vi "Read FPGA FIFO.vi"(6 "Error In":errorcluster, 9 "Vessel.lvclass":refnum<class "Vessel.lvclass">) -> (0 "Error Out":errorcluster, 3 "Vessel.lvclass 2":refnum<class "Vessel.lvclass">)   [LabVIEW 2014, in "Vessel.lvclass"]
uses:
  Vessel.lvclass
  Vessel.lvclass/Vessel.ctl
  <vilib>/Utility/error.llb/Error Cluster From Error Code.vi
  <vilib>/rvi/errors/niLvFpgaAdjustHostInterfaceError.vi
  <vilib>/rvi/interface/nirviMethod/nirviMethod.xnode
  FPGA Bitfiles/MinervaControlSy_FPGATarget_9870InterfaceDMA_4D1233B8.lvbitx
  cRIO/FPGA/9870 Interface DMA (FPGA).vi
  Supervisor/Supervisor.lvclass
  <vilib>/rvi/errors/niLvFpgaMergeErrorWithErrorCode.vi
  <vilib>/FPGAPlugInAG/cRIO-9074/niLvFpga_ReadFifo_cRIO-9074.vi
panel:
  in  "use chair":bool
  out "UDP error out":errorcluster
  out "APOS NED":dbl[](array[numeric]) format="%#.3f"
  out "kPa":dbl=100000.0 format="%#.1f"
  in  "depth ring":u16(ring)=2 items=["Saiv", "DVL", "Digiquartz"]
  out "DVL":string
  out "MT_BITS":u8[](array[numeric])
  out "Pos_s":dbl[](array[numeric])
  out "Altitudes":dbl[](array[numeric])
  out "Telebuf":u8[](array[numeric])
  out "NAVI OK":string
  out "MT_DATA":sgl[](array[numeric])
  in  "alt off [m]":dbl=0.2
  out "dvl_m":dbl[](array[numeric])
  out "MRU out":dbl[](array[numeric])
  out "Signals out":dbl[](array[numeric]) format="%#.2f"
  out "Elements Remaining\n after read":u32
  # "10."
  # "20."
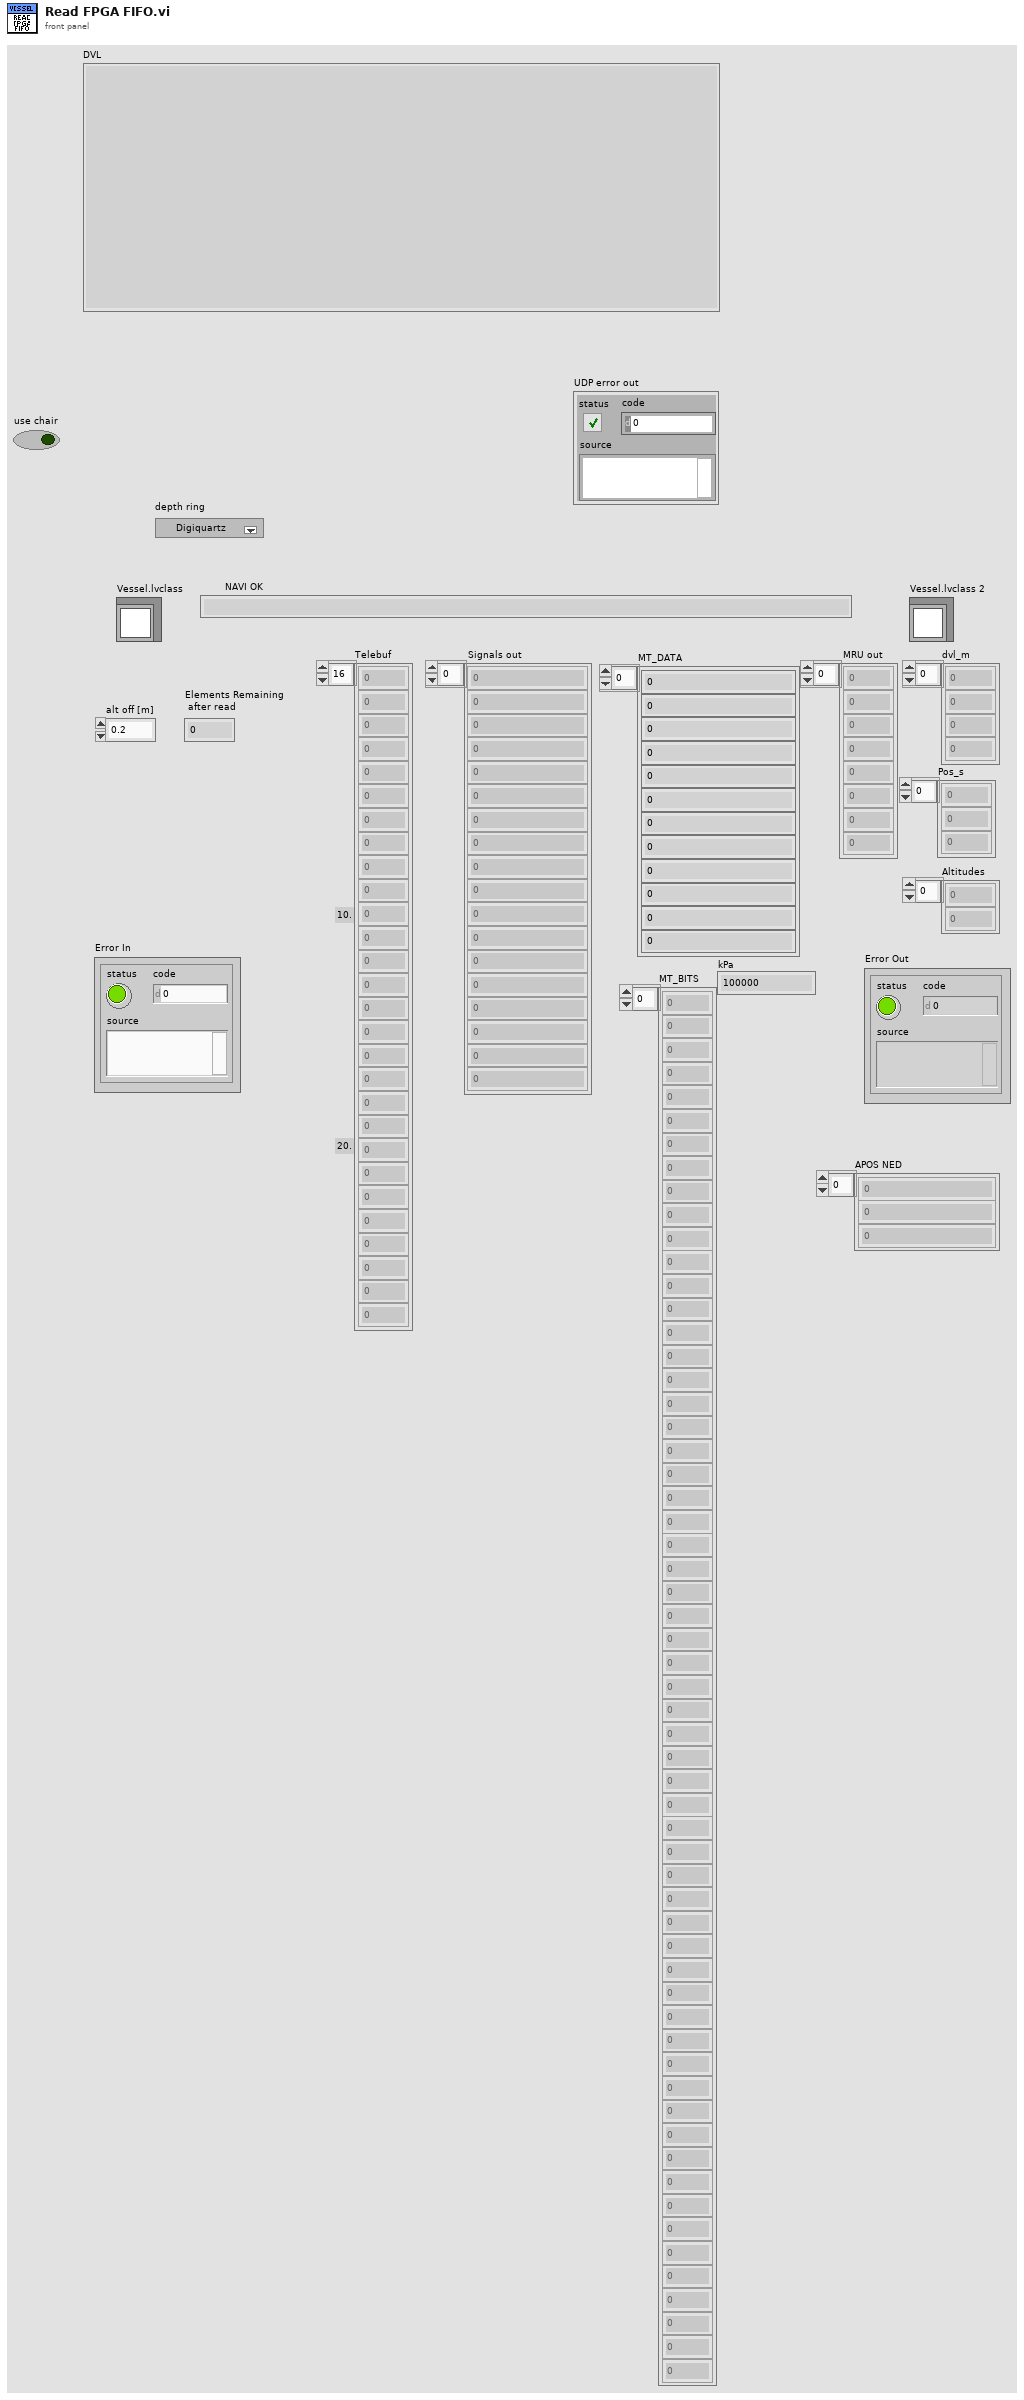
[diagram p1: front panel]
types:
  T1 = typedef "nicrio_cRIO-9871_BaudRateEnum.ctl" = enum16{"75 bps", "110 bps", "134 bps", "150 bps", "300 bps", "600 bps", "1200 bps", "1800 bps", "2400 bps", "4800 bps", "7200 bps", "9600 bps", "14.4 kbps", "19.2 kbps", "28.8 kbps", "38.4 kbps", "57.6 kbps", "115.2 kbps", "230.4 kbps", "460.8 kbps", "921.6 kbps"}
  T2 = typedef "nicrio_cRIO-9871_DataBitsEnum.ctl" = enum8{"5", "6", "7", "8"}
  T3 = typedef "nicrio_cRIO-9871_ParityEnum.ctl" = enum8{"None", "Odd", "Even", "Mark", "Space"}
  T4 = typedef "nicrio_cRIO-9871_StopBitsEnum.ctl" = enum8{"1", "1.5", "2"}
  T5 = typedef "nicrio_cRIO-9871_FlowControlEnum.ctl" = enum8{"None", "Software (XON / XOFF)", "Hardware (RTS / CTS)"}
  T6 = cluster{"Baud Rate":T1, "Data Bits":T2, "Parity":T3, "Stop Bits":T4, "Flow Control":T5}[]
  T7 = cluster{"Axis Translation":cluster{"X-Axis":dbl, "Y-Axis":dbl, "Z-Axis":dbl}, "Axis Rotation":cluster{"X-Axis":dbl, "Y-Axis":dbl, "Z-Axis":dbl}}
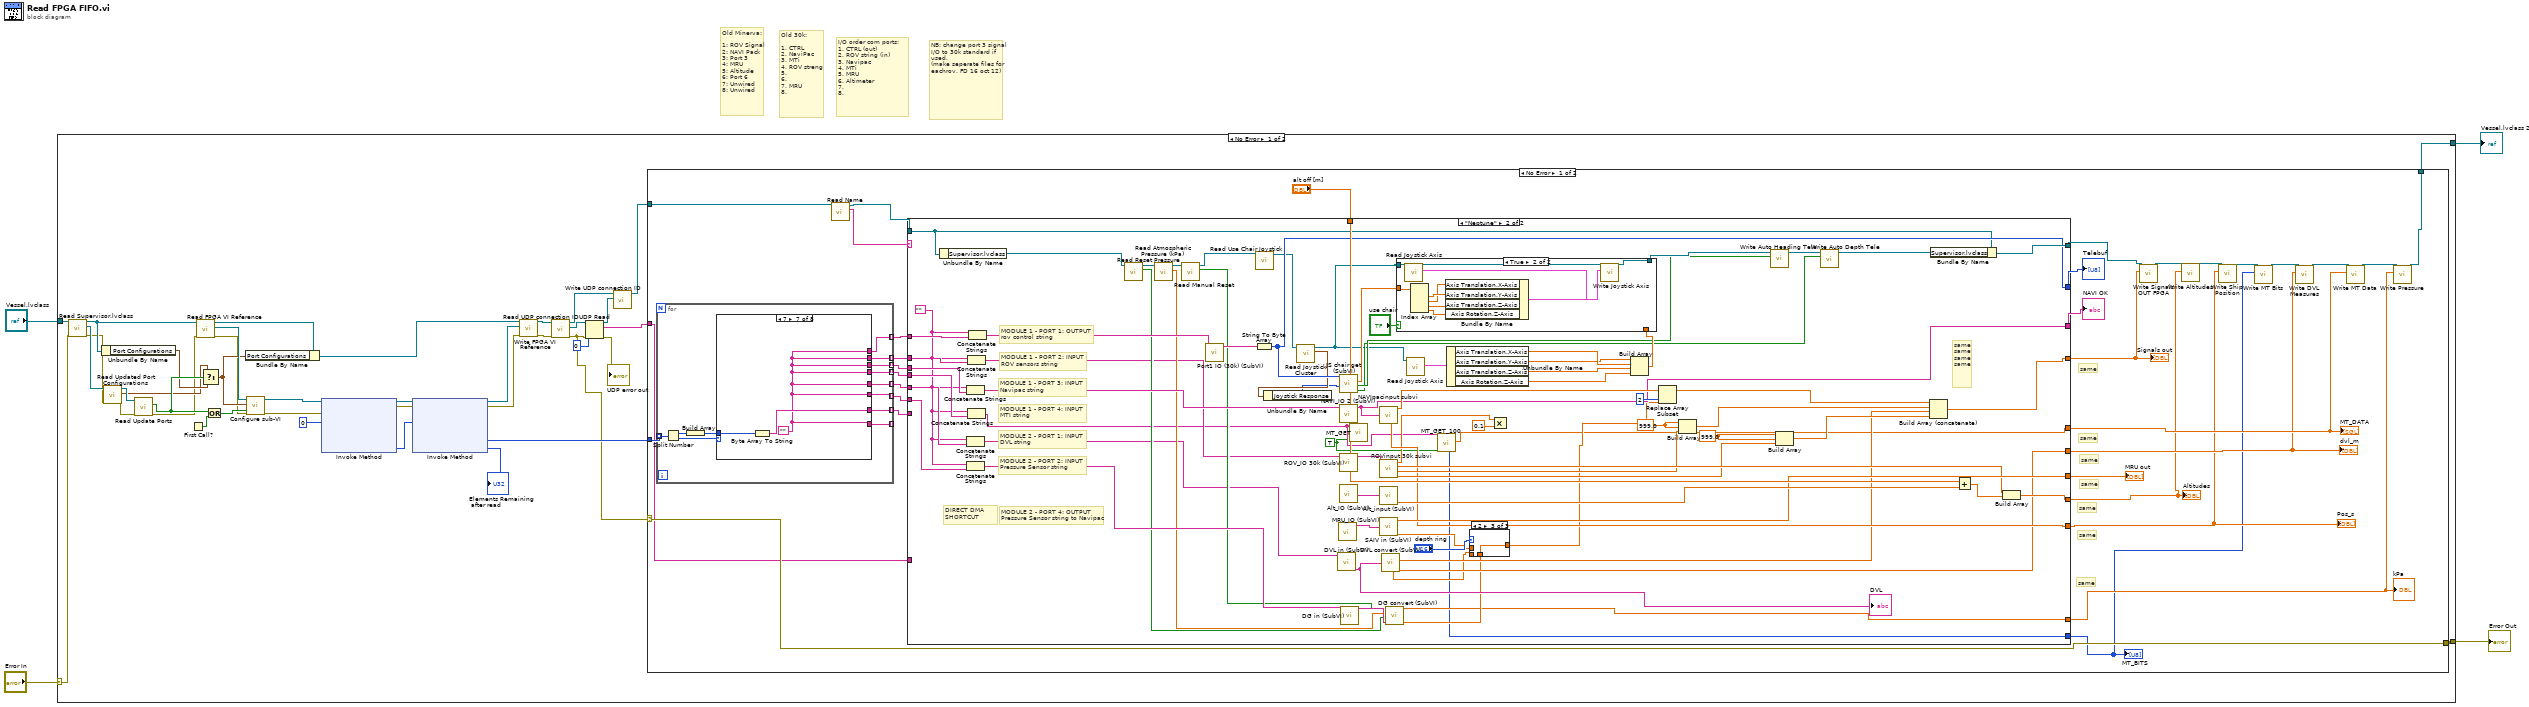
[diagram p0: block diagram]
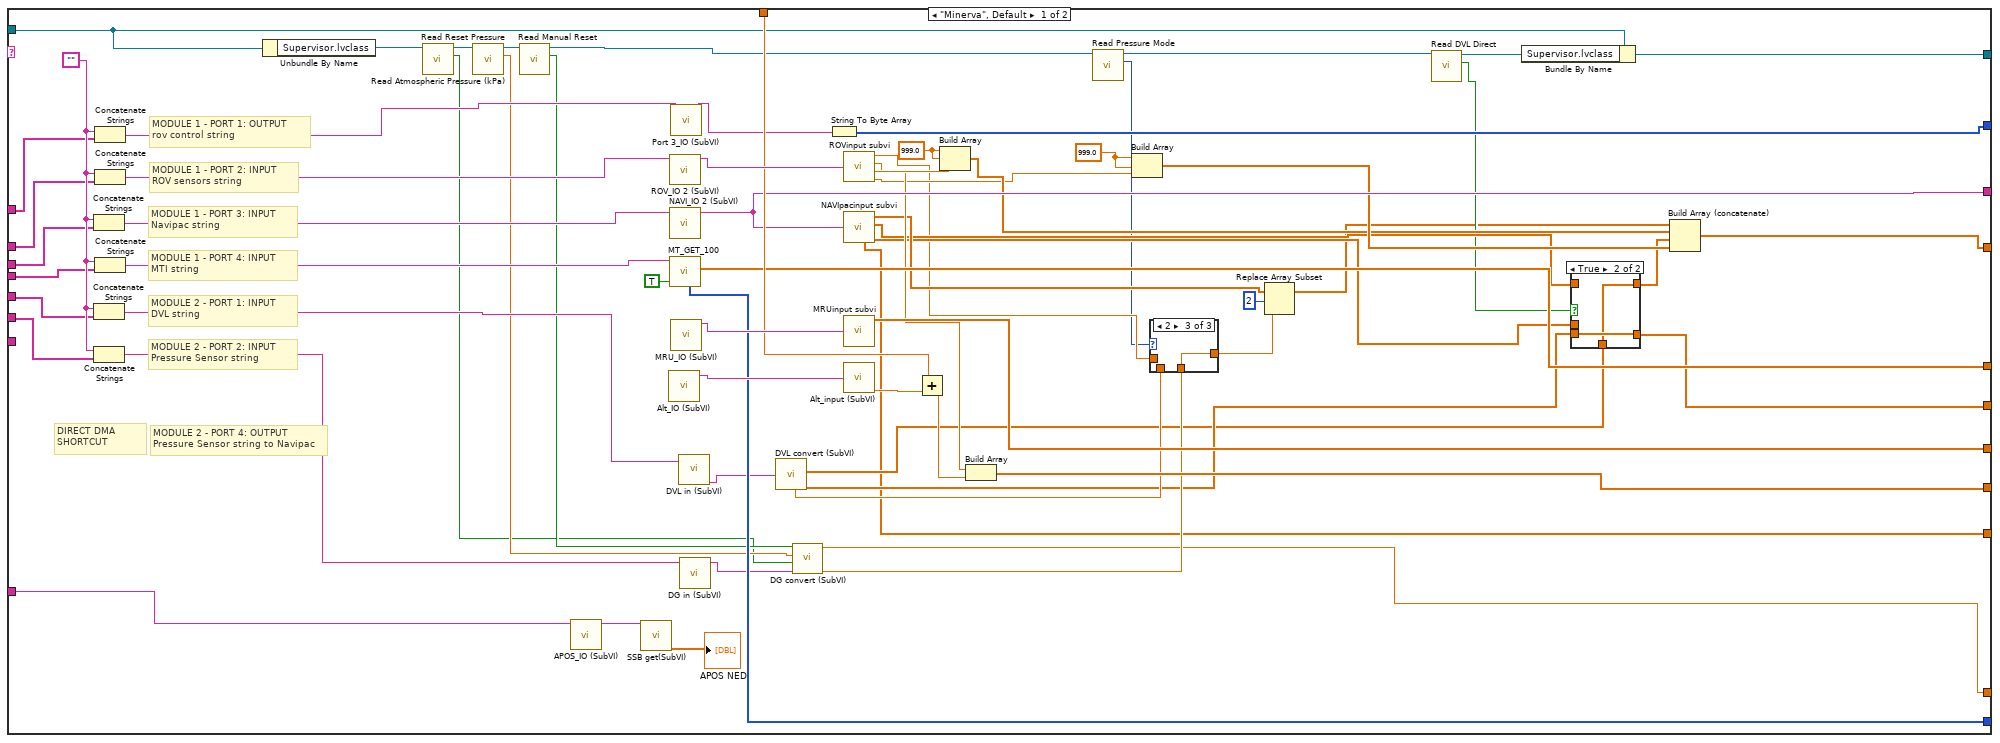
[diagram p2: hidden frame]
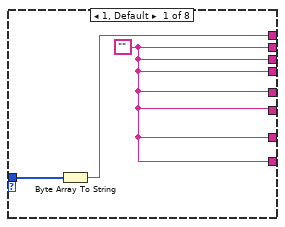
[diagram p9: hidden frame]
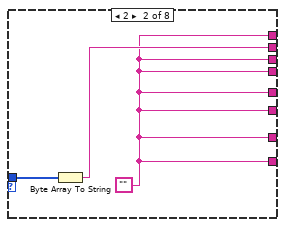
[diagram p10: hidden frame]
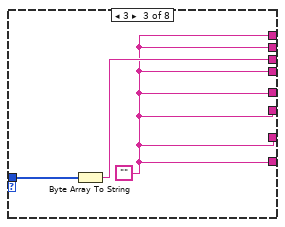
[diagram p11: hidden frame]
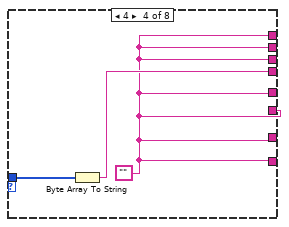
[diagram p12: hidden frame]
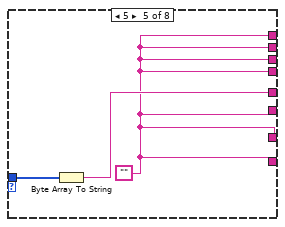
[diagram p13: hidden frame]
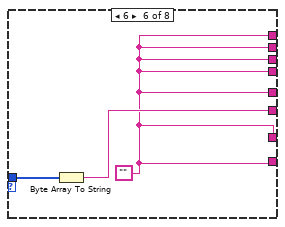
[diagram p14: hidden frame]
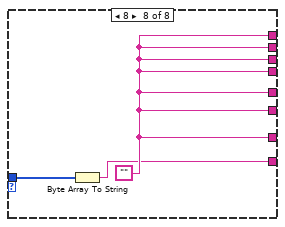
[diagram p15: hidden frame]
diagram:
  # "NB: change port 3 signal I/O to 30k standard if used. \n(make seperate files for eachrov, FD 16 oct 12)"
  # "I/O order com ports:\n1. CTRL (out)\n2. ROV string (in)\n3. Navipac\n4. MTi\n5. MRU\n6. Altimeter\n7. \n8."
  # "Old 30k:\n\n1. CTRL\n2. NaviPac\n3. MTi\n4. ROV streng\n5.\n6.\n7. MRU\n8."
  # "Old Minerva:\n\n1: ROV Signal\n2: NAVI Pack\n3: Port 3\n4: MRU\n5: Altitude \n6: Port 6\n7: Unwired\n8: Unwired"
  n1 = case shown="No Error" "Error In" {
    selector: "Error In" -> [w10 w281]
    tunnel: "Vessel.lvclass" -> [w33 w282]
    tunnel: [w36 w281] -> w2
    tunnel: [w22 w282] -> w1
    frame No Error {
      n2 = call "Read Supervisor.lvclass.vi"("error in (no error)"=w10, "Vessel in"=w33) -> ("error out"=w9:errorcluster, "Supervisor.lvclass"=w32:refnum<class "Supervisor.lvclass">, "Vessel out"=w28:refnum<class "Vessel.lvclass">)  [unwired: 7 in]
      n3 = Unbundle By Name(w28) -> ("Port Configurations"=w26:T6)
      n4 = call-dynamic "Read Updated Port Configurations.vi"("error in (no error)"=w9, "Supervisor in"=w32) -> ("error out"=w8:errorcluster, "Updated Port Configurations"=w25:T6, "Supervisor out"=w31:refnum<class "Supervisor.lvclass">)  [unwired: 7 in]
      n5 = call-dynamic "Read Update Ports.vi"("error in (no error)"=w8, "Supervisor in"=w31) -> ("error out"=w7:errorcluster, "Update Ports"=w27:bool)  [unwired: 7 in, 1 out]
      n6 = First Call?() -> (First Call?: T/F=w30:bool)
      n7 = call-dynamic "Read FPGA VI Reference.vi"("error in (no error)"=w7, "Vessel in"=w28) -> ("error out"=w6:errorcluster, "FPGA VI Reference Out"=w35:refnum<k20>, "Vessel out"=w24:refnum<class "Vessel.lvclass">)  [unwired: 7 in]
      n8 = Select(t=w25, s=w27, f=w26) -> (s? t:f=w23:T6)
      n9 = Or(x=w27, y=w30) -> (x .or. y?=w29:bool)
      n10 = Bundle By Name(cluster=w24, "Port Configurations"=w23) -> (w21:refnum<class "Vessel.lvclass">)
      n11 = call "Configure sub-VI.vi"("error in"=w6, "Update Config"=w29, "Port Configurations"=w23, "FPGA VI Reference In"=w35) -> ("error out"=w5:errorcluster, "FPGA VI Reference Out"=w34:refnum<k20>)  [unwired: 6 in]
      n12 = xnode "Invoke Method"("FPGA VI Reference In"=w34, "error in"=w5, "Number of Elements"=u32 0) -> ("FPGA VI Reference Out"=w41:refnum<k20>, "error out"=w42:errorcluster, "Elements Remaining"=w44:u32)  [unwired: 1 in, 1 out]
      n13 = xnode "Invoke Method"("FPGA VI Reference In"=w41, "error in"=w42, "Number of Elements"=w44) -> ("FPGA VI Reference Out"=w38:refnum<k20>, "error out"=w37:errorcluster, "Data"=w40:u16[], "Elements Remaining"=→"Elements Remaining\n after read":u32)  [unwired: 1 in]
      n14 = call-dynamic "Write FPGA VI Reference.vi"("error in (no error)"=w37, "FPGA VI Reference Out 2"=w38, "Vessel in"=w21) -> ("error out"=w18:errorcluster, "Vessel out"=w19:refnum<class "Vessel.lvclass">)  [unwired: 7 in]
      n15 = call-dynamic "Read UDP connection ID.vi"("error in (no error)"=w18, "Vessel in"=w19) -> ("error out"=w13:errorcluster, "UDP connection ID"=w20:refnum<k16>, "Vessel out"=w16:refnum<class "Vessel.lvclass">)  [unwired: 7 in]
      n16 = UDP Read(connection ID=w20, timeout ms (25000)=0, 8:w13) -> (data out=w17:string, error out=→"UDP error out":errorcluster, 3:w14:refnum<k16>)  [unwired: 1 in, 2 out]
      n17 = call-dynamic "Write UDP connection ID.vi"("UDP connection ID"=w14, "Vessel in"=w16) -> ("Vessel out"=w15:refnum<class "Vessel.lvclass">)  [unwired: 8 in, 1 out]
      n18 = case shown="No Error" w13 {
        selector: w13 -> [w71 w280]
        tunnel: w40 -> [w73 _]
        tunnel: [w71 w280] -> w36
        tunnel: w15 -> [w61 w279]
        tunnel: [w59 w279] -> w22
        tunnel: w17 -> [w60 _]
        frame No Error {
          # "same"
          # "same"
          # "same"
          # "same"
          # "same"
          # "same"
          # "same"
          n19 = for {
            tunnel: w73 -> [w248] mode=indexing
            tunnel: [w252] -> w74 mode=indexing
            tunnel: [w251] -> w75 mode=indexing
            tunnel: [w250] -> w69 mode=indexing
            tunnel: [w249] -> w76 mode=indexing
            tunnel: [w246] -> w72 mode=indexing
            tunnel: [w245] -> w68 mode=indexing
            tunnel: [w244] -> w67 mode=indexing
            tunnel: [w243] -> _ mode=indexing
            n20 = Split Number(x=w248) -> (hi(x)=w254:u8, lo(x)=w253:u8)
            n21 = Build Array(w254) -> (w247:u8[])
            n22 = case shown="7" w253 {
              tunnel: [w256 w258 w261 w264 w267 w270 w273 w277] -> w252
              tunnel: [w255 w259 w261 w264 w267 w270 w273 w277] -> w251
              tunnel: [w255 w258 w262 w264 w267 w270 w273 w277] -> w250
              tunnel: [w255 w258 w261 w265 w267 w270 w273 w277] -> w249
              tunnel: w247 -> [w257 w260 w263 w266 w269 w272 w275 w278]
              tunnel: [w255 w258 w261 w264 w268 w270 w273 w277] -> w246
              tunnel: [w255 w258 w261 w264 w267 w271 w273 w277] -> w245
              tunnel: [w255 w258 w261 w264 w267 w270 w274 w277] -> w244
              tunnel: [w255 w258 w261 w264 w267 w270 w273 w276] -> w243
              frame 1, Default {
                w255 = ""
                n23 = Byte Array To String(unsigned byte array=w257) -> (string=w256:string)
              }
              frame 2 {
                w258 = ""
                n24 = Byte Array To String(unsigned byte array=w260) -> (string=w259:string)
              }
              frame 3 {
                w261 = ""
                n25 = Byte Array To String(unsigned byte array=w263) -> (string=w262:string)
              }
              frame 4 {
                w264 = ""
                n26 = Byte Array To String(unsigned byte array=w266) -> (string=w265:string)
              }
              frame 5 {
                w267 = ""
                n27 = Byte Array To String(unsigned byte array=w269) -> (string=w268:string)
              }
              frame 6 {
                w270 = ""
                n28 = Byte Array To String(unsigned byte array=w272) -> (string=w271:string)
              }
              frame 7 {
                w273 = ""
                n29 = Byte Array To String(unsigned byte array=w275) -> (string=w274:string)
              }
              frame 8 {
                w277 = ""
                n30 = Byte Array To String(unsigned byte array=w278) -> (string=w276:string)
              }
            }
          }
          n31 = call-dynamic "Read Name.vi"("Vessel in"=w61) -> ("Name"=w65:string, "Vessel out"=w66:refnum<class "Vessel.lvclass">)  [unwired: 8 in, 1 out]
          n32 = case shown="\"Neptune\"" w65 {
            tunnel: w76 -> [w140 w228]
            tunnel: w75 -> [w142 w227]
            tunnel: w74 -> [w143 w226]
            tunnel: [w120 w186] -> w51
            tunnel: w72 -> [w139 w158]
            tunnel: [w131 w185] -> w70
            tunnel: [w101 w180] -> w54
            tunnel: w69 -> [w141 w222]
            tunnel: w68 -> [w138 w159]
            tunnel: w66 -> [w116 w195]
            tunnel: [w115 w219] -> w52
            tunnel: w67 -> [_ _]
            tunnel: "alt off [m]" -> [w132 w206]
            tunnel: [w130 w205] -> w63
            tunnel: [w127 w155] -> w56
            tunnel: [w128 w204] -> w62
            tunnel: [w117 w196] -> w45
            tunnel: [w79 w184] -> w53
            tunnel: [w113 w154] -> w48
            tunnel: [w95 w171] -> w58
            tunnel: w60 -> [w92 _]
            frame "Minerva", Default {
              w122 = 999.0 ("element")
              w124 = 999.0 ("element")
              w144 = ""
              # "DIRECT DMA SHORTCUT"
              # "MODULE 2 - PORT 4: OUTPUT\nPressure Sensor string to Navipac"
              # "MODULE 2 - PORT 2: INPUT\nPressure Sensor string"
              # "MODULE 2 - PORT 1: INPUT\nDVL string"
              # "MODULE 1 - PORT 4: INPUT\nMTI string"
              # "MODULE 1 - PORT 3: INPUT\nNavipac string"
              # "MODULE 1 - PORT 2: INPUT\nROV sensors string"
              # "MODULE 1 - PORT 1: OUTPUT\nrov control string"
              n33 = Concatenate Strings(w144, w141) -> (w126:string)
              n34 = Concatenate Strings(w144, w139) -> (w93:string)
              n35 = Concatenate Strings(w144, w138) -> (w107:string)
              n36 = Concatenate Strings(w144, w143) -> (w114:string)
              n37 = Concatenate Strings(w144, w142) -> (w94:string)
              n38 = Concatenate Strings(w144, w140) -> (w125:string)
              n39 = Unbundle By Name(w116) -> ("Supervisor.lvclass"=w84:refnum<class "Supervisor.lvclass">)
              n40 = call-dynamic "Read Reset Pressure.vi"("Supervisor in"=w84) -> ("Reset Pressure"=w81:bool, "Supervisor out"=w86:refnum<class "Supervisor.lvclass">)  [unwired: 8 in, 1 out]
              n41 = call-dynamic "Read Atmospheric Pressure (kPa).vi"("Supervisor in"=w86) -> ("Atmospheric Pressure (deciBar)"=w82:dbl, "Supervisor out"=w85:refnum<class "Supervisor.lvclass">)  [unwired: 8 in, 1 out]
              n42 = call-dynamic "Read Manual Reset.vi"("Supervisor in"=w85) -> ("Manual Reset"=w83:bool, "Supervisor out"=w77:refnum<class "Supervisor.lvclass">)  [unwired: 8 in, 1 out]
              n43 = call "APOS_IO (SubVI).vi"("GPS in"=w92) -> ("GPS OK"=w91:string)  [unwired: 9 in, 1 out]
              n44 = call "SSB get(SubVI).vi"("String"=w91) -> ("APOS NED"=→"APOS NED":dbl[])  [unwired: 4 in, 1 out]
              n45 = call "Alt_IO (SubVI).vi"() -> ("Altimeter OK"=w135:string)  [unwired: 11 in]
              n46 = call "ROV_IO 2 (SubVI).vi"("ROV string"=w94) -> ("ROV OK"=w137:string)  [unwired: 10 in]
              n47 = call "NAVI_IO 2 (SubVI).vi"("NAVI string"=w126) -> ("NAVI OK"=w131:string)  [unwired: 10 in]
              n48 = call "MT_GET_100.vi"("Use checksum"=TRUE, "read buffer"=w125) -> ("MT_DATA"=w127:sgl[], "MT_BITS"=w113:u8[])  [unwired: 6 in, 2 out]
              n49 = call "Port 3_IO (SubVI).vi"("port 3 hex  string"=w114) -> ("port 3 OK"=w129:string)  [unwired: 10 in]
              n50 = call "MRU_IO (SubVI).vi"() -> ("MRU OK"=w134:string)  [unwired: 11 in]
              n51 = call "DVL in (SubVI).vi"("DVL string"=w93) -> ("DVL OK"=w111:string)  [unwired: 10 in]
              n52 = call "DG in (SubVI).vi"("DG string"=w107) -> ("DG OK"=w112:string)  [unwired: 10 in]
              n53 = call "DVL convert (SubVI).vi"("String"=w111) -> ("depth"=w105:dbl, "dvl alts"=w102:dbl[], "u_bt_dvl"=w97:dbl[])  [unwired: 1 in, 2 out]
              n54 = call "DG convert (SubVI).vi"("String"=w112, "Reset pressure"=w81, "atm kPa"=w82, "manual reset"=w83) -> ("depth"=w104:dbl, "Pressure (deciBAR = 10*kPASCAL)"=w95:dbl)  [unwired: 1 in, 1 out]
              n55 = String To Byte Array(string=w129) -> (unsigned byte array=w128:u8[])
              n56 = call "ROVinput subvi.vi"("String"=w137) -> ("depth"=w96:dbl, "altitude"=w119:dbl, "heading"=w123:dbl, "yaw rate"=w106:dbl)
              n57 = call "NAVIpacinput subvi.vi"("String"=w131) -> ("Pos_s"=w79:dbl[], "a_dvl"=w100:dbl[], "vb_dvl"=w99:dbl[], "NED_tp"=w110:dbl[])  [unwired: 2 out]
              n58 = call "MRUinput subvi.vi"("String"=w134) -> ("MRU out"=w130:dbl[])  [unwired: 3 in]
              n59 = call "Alt_input (SubVI).vi"("String"=w135) -> ("altitude"=w133:dbl)  [unwired: 3 in]
              n60 = Add(x=w132, y=w133) -> (x+y=w118:dbl)
              n61 = Build Array(w124, w124, w123) -> (w108:dbl[])
              n62 = Build Array(w119, w118) -> (w117:dbl[])
              n63 = call-dynamic "Read Pressure Mode.vi"("Supervisor in"=w77) -> ("Pressure Mode"=w87:i16, "Supervisor out"=w80:refnum<class "Supervisor.lvclass">)  [unwired: 8 in, 1 out]
              n64 = Build Array(w122, w122, w106) -> (w121:dbl[])
              n65 = case shown="2" w87 {
                tunnel: w105 -> [_ w150 _]
                tunnel: [w149 w150 w151] -> w103
                tunnel: w96 -> [w149 _ _]
                tunnel: w104 -> [_ _ w151]
                frame 0, Default {
                }
                frame 1 {
                }
                frame 2 {
                }
              }
              n66 = Replace Array Subset(array=w110, new element=w103, index=2) -> (w78:dbl[])
              n67 = call-dynamic "Read DVL Direct.vi"("Supervisor in"=w80) -> ("DVL Direct"=w88:bool, "Supervisor out"=w89:refnum<class "Supervisor.lvclass">)  [unwired: 8 in, 1 out]
              n68 = Bundle By Name(cluster=w116, "Supervisor.lvclass"=w89) -> (w115:refnum<class "Vessel.lvclass">)
              n69 = case shown="True" w88 {
                tunnel: w102 -> [_ w148]
                tunnel: [w146 w148] -> w101
                tunnel: w100 -> [w146 _]
                tunnel: w99 -> [w145 _]
                tunnel: [w145 w147] -> w98
                tunnel: w97 -> [_ w147]
                frame False {
                }
                frame True {
                }
              }
              n70 = Build Array (concatenate)(w78, w108, w98, w121) -> (w120:dbl[])
            }
            frame "Neptune" {
              w189 = 999.0 ("element")
              w160 = 999.0 ("element")
              w156 = TRUE ("Use checksum")
              w152 = ""
              # "DIRECT DMA SHORTCUT"
              # "MODULE 2 - PORT 4: OUTPUT\nPressure Sensor string to Navipac"
              # "MODULE 2 - PORT 2: INPUT\nPressure Sensor string"
              # "MODULE 2 - PORT 1: INPUT\nDVL string"
              # "MODULE 1 - PORT 4: INPUT\nMTI string"
              # "MODULE 1 - PORT 3: INPUT\nNavipac string"
              # "MODULE 1 - PORT 2: INPUT\nROV sensors string"
              # "MODULE 1 - PORT 1: OUTPUT\nrov control string"
              # "same\nsame\nsame\nsame"
              n71 = Unbundle By Name(w195) -> ("Supervisor.lvclass"=w168:refnum<class "Supervisor.lvclass">)
              n72 = Concatenate Strings(w152, w222) -> (w199:string)
              n73 = Concatenate Strings(w152, w158) -> (w161:string)
              n74 = Concatenate Strings(w152, w159) -> (w173:string)
              n75 = Concatenate Strings(w152, w227) -> (w162:string)
              n76 = Concatenate Strings(w152, w228) -> (w157:string)
              n77 = Concatenate Strings(w152, w226) -> (w221:string)
              n78 = call-dynamic "Read Reset Pressure.vi"("Supervisor in"=w168) -> ("Reset Pressure"=w164:bool, "Supervisor out"=w170:refnum<class "Supervisor.lvclass">)  [unwired: 8 in, 1 out]
              n79 = call-dynamic "Read Atmospheric Pressure (kPa).vi"("Supervisor in"=w170) -> ("Atmospheric Pressure (deciBar)"=w165:dbl, "Supervisor out"=w169:refnum<class "Supervisor.lvclass">)  [unwired: 8 in, 1 out]
              n80 = call-dynamic "Read Manual Reset.vi"("Supervisor in"=w169) -> ("Manual Reset"=w166:bool, "Supervisor out"=w167:refnum<class "Supervisor.lvclass">)  [unwired: 8 in, 1 out]
              n81 = call "Port1 IO (30k) (SubVI).vi"("port 3 hex  string"=w221) -> ("port 3 OK"=w220:string)  [unwired: 10 in]
              n82 = String To Byte Array(string=w220) -> (unsigned byte array=w204:u8[])
              n83 = call-dynamic "Read Use Chair Joystick.vi"("Supervisor in"=w167) -> ("Supervisor out"=w203:refnum<class "Supervisor.lvclass">)  [unwired: 8 in, 2 out]
              n84 = call-dynamic "Read Joystick Cluster.vi"("Supervisor in"=w203) -> ("Joystick Cluster"=w202:cluster{"Joystick Response":u16}, "Supervisor out"=w201:refnum<class "Supervisor.lvclass">)  [unwired: 8 in, 1 out]
              n85 = Unbundle By Name(w202) -> ("Joystick Response"=w200:u16)
              n86 = call "DVL in (SubVI).vi"("DVL string"=w161) -> ("DVL OK"=w179:string)  [unwired: 10 in]
              "DVL" <- w179
              n87 = call "MRU_IO (SubVI).vi"() -> ("MRU OK"=w225:string)  [unwired: 11 in]
              n88 = call "JS chair get (SubVI).vi"("JS resp"=w200, "Telebuf in"=w204) -> ("Auto Depth"=w208:bool, "Auto Heading"=w209:bool, "t_js_prc"=w212:dbl[])  [unwired: 6 in, 1 out]
              n89 = call "NAVI_IO 2 (SubVI).vi"("NAVI string"=w199) -> ("NAVI OK"=w185:string)  [unwired: 10 in]
              n90 = call "ROV_IO 30k (SubVI).vi"("ROV string"=w162) -> ("ROV OK"=w207:string)  [unwired: 10 in]
              n91 = call "Alt_IO (SubVI).vi"() -> ("Altimeter OK"=w224:string)  [unwired: 11 in]
              n92 = call "DG in (SubVI).vi"("DG string"=w173) -> ("DG OK"=w178:string)  [unwired: 10 in]
              n93 = call "MT_GET.vi"("Use checksum"=w156, "read buffer"=w157) -> ()  [unwired: 6 in, 4 out]
              n94 = call "NAVIpacinput subvi.vi"("String"=w185) -> ("Pos_s"=w184:dbl[], "NED_tp"=w194:dbl[])  [unwired: 4 out]
              n95 = call "ROVinput 30k subvi.vi"("String"=w207) -> ("depth"=w182:dbl, "altitude"=w198:dbl, "heading"=w191:dbl, "yaw rate"=w188:dbl)
              n96 = call "Alt_input (SubVI).vi"("String"=w224) -> ("altitude"=w223:dbl)  [unwired: 3 in]
              n97 = call "SAIV in (SubVI).vi"("String"=w225) -> ("SAIV out"=w205:dbl[], "depth"=w174:dbl)  [unwired: 2 in]
              n98 = call "DVL convert (SubVI).vi"("String"=w179) -> ("depth"=w176:dbl, "dvl alts"=w180:dbl[], "u_bt_dvl"=w181:dbl[])  [unwired: 1 in, 2 out]
              n99 = call "DG convert (SubVI).vi"("String"=w178, "Reset pressure"=w164, "atm kPa"=w165, "manual reset"=w166) -> ("depth"=w172:dbl, "Pressure (deciBAR = 10*kPASCAL)"=w171:dbl)  [unwired: 1 in, 1 out]
              n100 = call-dynamic "Read Joystick Axis.vi"("Supervisor in"=w201) -> ("Joystick Axis"=w218:T7)  [unwired: 8 in, 2 out]
              n101 = call "MT_GET_100.vi"("Use checksum"=w156, "read buffer"=w157) -> ("MT_DATA"=w155:sgl[], "MT_BITS"=w154:u8[])  [unwired: 6 in, 2 out]
              n102 = Unbundle By Name(w218) -> ("Axis Translation.X-Axis"=w217:dbl, "Axis Translation.Y-Axis"=w216:dbl, "Axis Translation.Z-Axis"=w215:dbl, "Axis Rotation.Z-Axis"=w214:dbl)
              n103 = case shown="2" "depth ring" {
                tunnel: w176 -> [_ w230 _]
                tunnel: [w229 w230 w231] -> w175
                tunnel: w174 -> [w229 _ _]
                tunnel: w172 -> [_ _ w231]
                frame 0, Default {
                }
                frame 1 {
                }
                frame 2 {
                }
              }
              n104 = Multiply(x=w182, y=0.1) -> ()  [unwired: 1 out]
              n105 = Build Array(w216, w217, w215, w214) -> (w213:dbl[])
              n106 = case shown="True" "use chair" {
                tunnel: w212 -> [_ w239]
                tunnel: w201 -> [w232 w242]
                tunnel: [w232 w234] -> w211
                tunnel: w213 -> [_ _]
                frame False {
                }
                frame True {
                  n107 = call-dynamic "Read Joystick Axis.vi"("Supervisor in"=w242) -> ("Joystick Axis"=w233:T7, "Supervisor out"=w241:refnum<class "Supervisor.lvclass">)  [unwired: 8 in, 1 out]
                  n108 = Index Array(array=w239) -> (element #1=w238:dbl, element #2=w237:dbl, element #3=w236:dbl, element #4=w235:dbl)  [unwired: 4 in]
                  n109 = Bundle By Name(cluster=w233, "Axis Translation.X-Axis"=w237, "Axis Translation.Y-Axis"=w238, "Axis Translation.Z-Axis"=w236, "Axis Rotation.Z-Axis"=w235) -> (w240:T7)
                  n110 = call-dynamic "Write Joystick Axis.vi"("Joystick Axis"=w240, "Supervisor in"=w241) -> ("Supervisor out"=w234:refnum<class "Supervisor.lvclass">)  [unwired: 8 in, 1 out]
                }
              }
              n111 = Replace Array Subset(array=w194, new element=w175, index=2) -> (w192:dbl[])
              n112 = Build Array(w160, w160, w191) -> (w190:dbl[])
              n113 = call-dynamic "Write Auto Heading Tele.vi"("Auto Heading Tele"=w209, "Supervisor in"=w211) -> ("Supervisor out"=w210:refnum<class "Supervisor.lvclass">)  [unwired: 8 in, 1 out]
              n114 = Build Array(w189, w189, w188) -> (w187:dbl[])
              n115 = call-dynamic "Write Auto Depth Tele.vi"("Auto Depth Tele"=w208, "Supervisor in"=w210) -> ("Supervisor out"=w163:refnum<class "Supervisor.lvclass">)  [unwired: 8 in, 1 out]
              n116 = Build Array (concatenate)(w192, w190, w181, w187) -> (w186:dbl[])
              n117 = Bundle By Name(cluster=w195, "Supervisor.lvclass"=w163) -> (w219:refnum<class "Vessel.lvclass">)
              n118 = Add(x=w206, y=w223) -> (x+y=w197:dbl)
              n119 = Build Array(w198, w197) -> (w196:dbl[])
            }
          }
          "Signals out" <- w51
          "dvl_m" <- w54
          "NAVI OK" <- w70
          "MRU out" <- w63
          "MT_DATA" <- w56
          "Telebuf" <- w62
          "Altitudes" <- w45
          "Pos_s" <- w53
          "MT_BITS" <- w48
          "kPa" <- w58
          n120 = call-dynamic "Write Signals OUT FPGA.vi"("Signals OUT"=w51, "Vessel in"=w52) -> ("Vessel out"=w47:refnum<class "Vessel.lvclass">)  [unwired: 8 in, 1 out]
          n121 = call-dynamic "Write Altitudes.vi"("Altitudes"=w45, "Vessel in"=w47) -> ("Vessel out"=w46:refnum<class "Vessel.lvclass">)  [unwired: 8 in, 1 out]
          n122 = call-dynamic "Write Ship Position.vi"("Ship Position"=w53, "Vessel in"=w46) -> ("Vessel out"=w49:refnum<class "Vessel.lvclass">)  [unwired: 8 in, 1 out]
          n123 = call-dynamic "Write MT Bits.vi"("MT Bits"=w48, "Vessel in"=w49) -> ("Vessel out"=w50:refnum<class "Vessel.lvclass">)  [unwired: 8 in, 1 out]
          n124 = call-dynamic "Write DVL Measures.vi"("DVL Measures"=w54, "Vessel in"=w50) -> ("Vessel out"=w55:refnum<class "Vessel.lvclass">)  [unwired: 8 in, 1 out]
          n125 = call-dynamic "Write MT Data.vi"("MT Data"=w56, "Vessel in"=w55) -> ("Vessel out"=w57:refnum<class "Vessel.lvclass">)  [unwired: 8 in, 1 out]
          n126 = call-dynamic "Write Pressure.vi"("Pressure"=w58, "Vessel in"=w57) -> ("Vessel out"=w59:refnum<class "Vessel.lvclass">)  [unwired: 8 in, 1 out]
        }
        frame Error {
        }
      }
    }
    frame Error {
    }
  }
  "Vessel.lvclass 2" <- w1
  "Error Out" <- w2
